vi "Ramp Up Voltage.vi"(11 "VISA Refnum in":refnum<visa-resource-name>) -> (0 "error out":errorcluster, 2 "BoardHandle out":T1)   [LabVIEW 2020]
uses:
  <instrlib>/CAEN PSM/CAEN PSM.lvlib
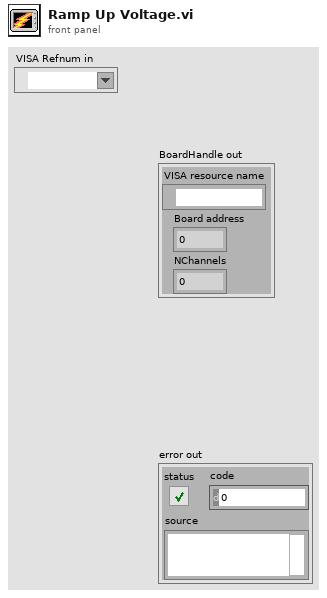
[diagram p1: front panel]
types:
  T1 = cluster{"VISA resource name":refnum<visa-resource-name>, "Board address":u8, "NChannels":u8}
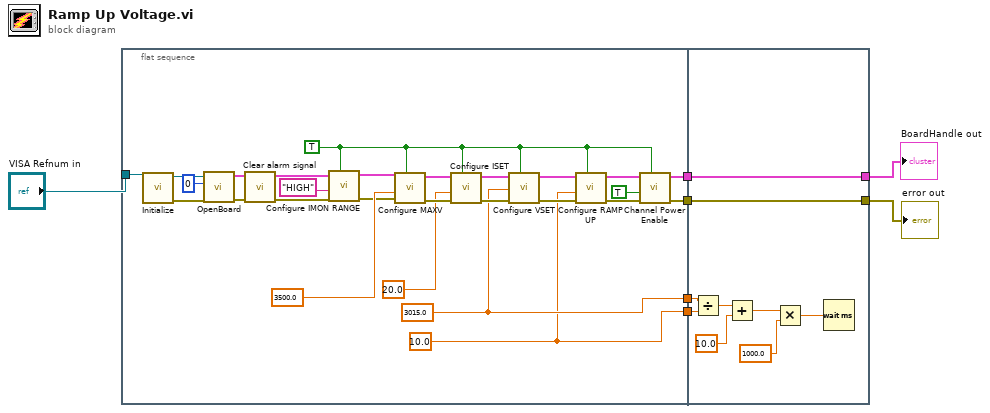
[diagram p0: block diagram]
diagram:
  n1 = flat-sequence {
    tunnel: [w20] -> w7
    tunnel: [w19] -> w6
    tunnel: [w18] -> w5
    tunnel: [w17] -> w4
    tunnel: "VISA Refnum in" -> [w16]
    tunnel: w7 -> [w38]
    tunnel: w6 -> [w37]
    tunnel: [w36] -> w3
    tunnel: w5 -> [w36]
    tunnel: [w35] -> w2
    tunnel: w4 -> [w35]
    frame #0 {
      w9 = TRUE ("All Channels (F)")
      w20 = 3015.0 ("Voltage Set (Volts)")
      w19 = 10.0 ("Voltage Ramp Up (V/s)")
      n2 = call <instrlib>:"Initialize.vi"("VISA resource name"=w16) -> ("error out"=w29:errorcluster, "VISA resource name out"=w26:refnum<visa-resource-name>)  [unwired: 9 in]
      n3 = call <instrlib>:"OpenBoard.vi"("error in (no error)"=w29, "Board Address"=u8 0, "VISA resource name"=w26) -> ("error out"=w30:errorcluster, "BoardHandle"=w25:T1)  [unwired: 7 in]
      n4 = call <instrlib>:"Clear alarm signal.vi"("error in (no error)"=w30, "BoardHandle"=w25) -> ("error out"=w14:errorcluster, "BoardHandle out"=w13:T1)  [unwired: 8 in]
      n5 = call <instrlib>:"Configure IMON RANGE.vi"("All Channels (F)"=w9, "error in (no error)"=w14, "IMon range (LOW)"="HIGH", "BoardHandle"=w13) -> ("error out"=w10:errorcluster, "BoardHandle out"=w11:T1)  [unwired: 6 in]
      n6 = call <instrlib>:"Configure MAXV.vi"("All Channels (F)"=w9, "error in (no error)"=w10, "Voltage Max (0.0 V)"=3500.0 ("VMax (Volts)"), "BoardHandle"=w11) -> ("error out"=w31:errorcluster, "BoardHandle out"=w24:T1)  [unwired: 6 in]
      n7 = call <instrlib>:"Configure ISET.vi"("All Channels (F)"=w9, "error in (no error)"=w31, "Current Limit (0.00 uA)"=20.0 ("Current Limit (uA)"), "BoardHandle"=w24) -> ("error out"=w32:errorcluster, "BoardHandle out"=w23:T1)  [unwired: 6 in]
      n8 = call <instrlib>:"Configure VSET.vi"("All Channels (F)"=w9, "error in (no error)"=w32, "Voltage Level (0.0 V)"=w20, "BoardHandle"=w23) -> ("error out"=w33:errorcluster, "BoardHandle out"=w22:T1)  [unwired: 6 in]
      n9 = call <instrlib>:"Configure RAMP UP.vi"("All Channels (F)"=w9, "error in (no error)"=w33, "Voltage ramp up (0 V/s)"=w19, "BoardHandle"=w22) -> ("error out"=w34:errorcluster, "BoardHandle out"=w21:T1)  [unwired: 6 in]
      n10 = call <instrlib>:"Channel Power Enable.vi"("All Channels (F)"=w9, "error in (no error)"=w34, "Enable (OFF)"=TRUE ("Boolean"), "BoardHandle"=w21) -> ("error out"=w17:errorcluster, "BoardHandle out"=w18:T1)  [unwired: 6 in]
    }
    frame #1 {
      n11 = Divide(x=w38, y=w37) -> (x/y=w41:dbl)
      n12 = Add(x=w41, y=10.0) -> (x+y=w42:dbl)
      n13 = Multiply(x=w42, y=1000.0) -> (x*y=w43:dbl)
      n14 = Wait (ms)(milliseconds to wait=w43) -> ()  [unwired: 1 out]
    }
  }
  "BoardHandle out" <- w3
  "error out" <- w2
